vi "DeleteSelectRowTable.vi"(8 "エラー入力":errorcluster, 9 "削除する長さ":i32, 10 "削除する指定行":i32, 11 "Tbl refnum":refnum<vi>) -> (0 "エラー出力":errorcluster, 3 "リファレンス出力":refnum<vi>)   [LabVIEW 2014]
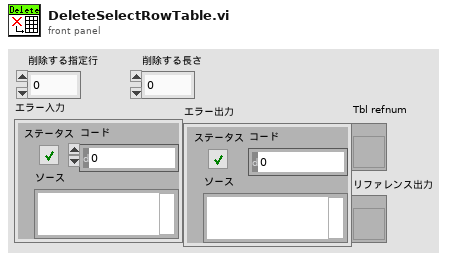
[diagram p1: front panel]
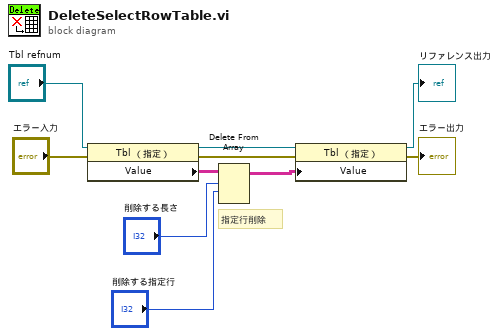
[diagram p0: block diagram]
diagram:
  # "指定行削除"
  n1 = property class="Tbl （指定）"(reference="Tbl refnum", error in="エラー入力") -> (reference out=w3:refnum<vi>, error out=w2:errorcluster, "Value"=w8:string[][])
  n2 = Delete From Array(array=w8, length="削除する長さ", index (row)="削除する指定行") -> (array with subset deleted=w4:string[][])  [unwired: 1 in, 1 out]
  n3 = property class="Tbl （指定）"(reference=w3, error in=w2, "Value"=w4) -> (reference out=→"リファレンス出力":refnum<vi>, error out=→"エラー出力":errorcluster)
